vi "tipshaping.action.vi"(8 "Error in (no error)":errorcluster, 10 "Application reference":refnum<vi>, 11 "TipShapingParam":T1={"TipLift"=-1.8e-09, "Bias Settling Time"=0.2, "Lift Height"=-3.6e-09, "Lift Time 2"=0.2, "Lifting Bias"=0.02, "Lift Time 1"=0.2} {"Lift Time 1" min=0.02 max=600.0 format="%.2p"; "Lifting Bias" format="%.3p"; "Lift Time 2" min=0.02 max=600.0 format="%.2p"; "Lift Height" format="%.2p"; "Bias Settling Time" format="%.2p"; "TipLift" format="%.2p"}) -> (0 "error out":errorcluster, 2 "Application ref out":refnum<vi>, 3 "dz":sgl=-5.693078e-09)   [LabVIEW 2014]
uses:
  <userlib>/Nanonis Prog Interface V5/Nanonis Prog Interface.lvlib
panel:
  out "z channel":i32=30
  out "initialz":sgl=-5.016415e-08 format="%#_6p"
  in  "Feedback":bool=TRUE
  in  "Switch Gain":bool
  in  "Current Gain":u16(ring) items=["HS 10^5", "HS 10^6", "HS 10^7", "HS 10^8", "HS 10^9", "HS 10^10", "HS 10^11", "LN 10^3", "LN 10^4", "LN 10^5", "LN 10^6", "LN 10^7", "LN 10^8", "LN 10^9"]
  in  "Bias value":dbl=1.0 format="%.3p"
  in  "Change Bias":bool
  out "Lift Time 1":dbl=0.2 min=0.02 max=600.0 format="%.2p"
  in  "End Wait Time":dbl=0.1 format="%.2p"
  out "Lifting Bias":dbl=-8.0 format="%.3p"
  out "Lift Time 2":dbl=0.2 min=0.02 max=600.0 format="%.2p"
  out "Lift Height":dbl format="%.2p"
  out "Bias Settling Time":dbl=0.2 format="%.2p"
  out "TipLift":dbl format="%.2p"
  in  "Switch Off Delay":dbl=0.1 format="%.2p"
  out "allQuit":bool
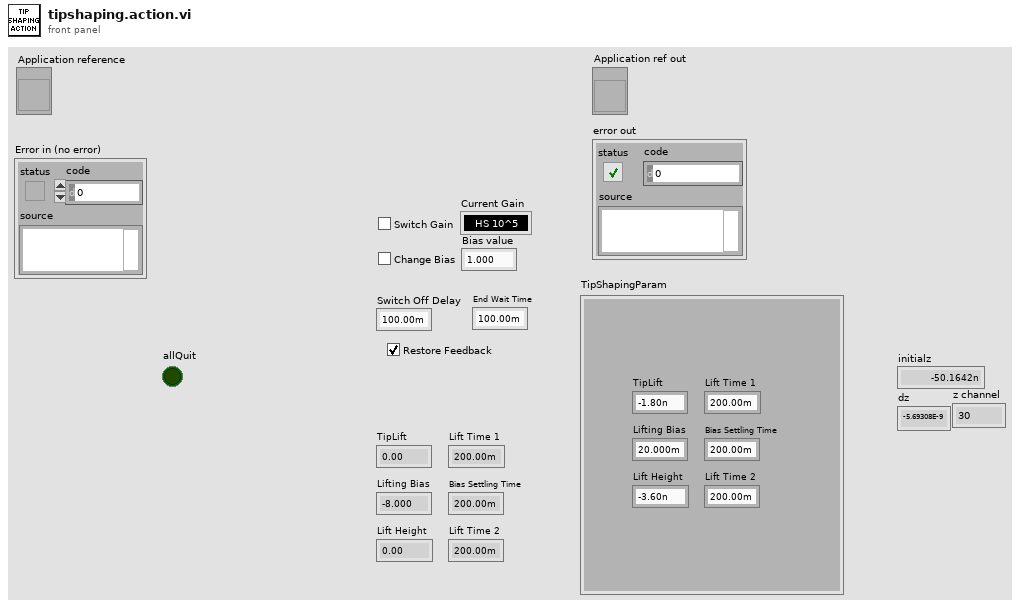
[diagram p1: front panel]
types:
  T1 = cluster{"TipLift":dbl, "Bias Settling Time":dbl, "Lift Height":dbl, "Lift Time 2":dbl, "Lifting Bias":dbl, "Lift Time 1":dbl}
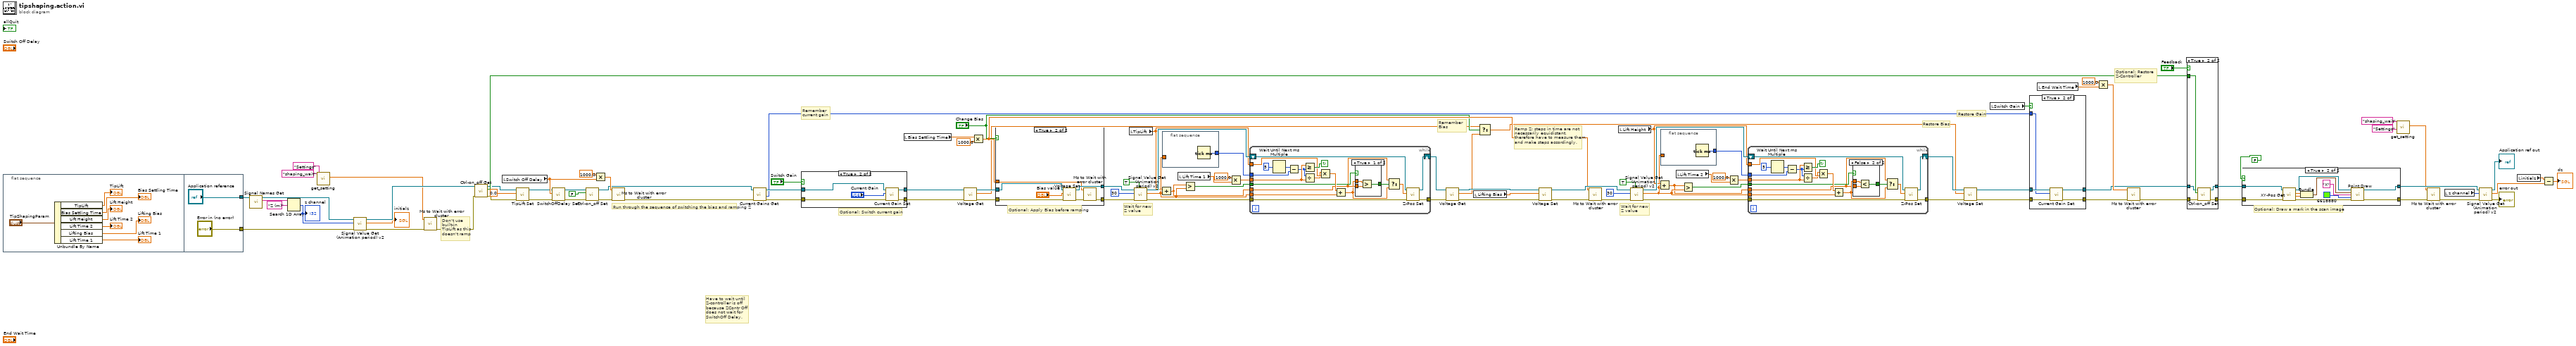
[diagram p0: block diagram]
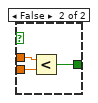
[diagram p6: hidden frame]
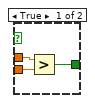
[diagram p8: hidden frame]
diagram:
  # "Ramp Z: steps in time are not necessarily equidistant, therefore have to measure them and make steps accordingly."
  # "Optional: Draw a mark in the scan image"
  # "Optional: Apply Bias before ramping"
  # "Remember Bias"
  # "Optional: Switch current gain"
  # "Remember current gain"
  # "Restore Bias"
  # "Optional: Restore Z-Controller"
  # "Restore Gain"
  # "Don't use built-in TipLift as this doesn't ramp"
  # "Wait for new Z value"
  # "Have to wait until Z-controller is off because ZContr Off does not wait for SwitchOff Delay."
  # "Wait for new Z value"
  # "Run through the sequence of switching the bias and ramping Z"
  n1 = flat-sequence {
    tunnel: ["Application reference"] -> w15
    tunnel: ["Error in (no error)"] -> w14
    frame #0 {
      n2 = Unbundle By Name("TipShapingParam") -> ("TipLift"=→"TipLift":dbl, "Bias Settling Time"=→"Bias Settling Time":dbl, "Lift Height"=→"Lift Height":dbl, "Lift Time 2"=→"Lift Time 2":dbl, "Lifting Bias"=→"Lifting Bias":dbl, "Lift Time 1"=→"Lift Time 1":dbl)
    }
    frame #1 {
    }
  }
  n3 = call <userlib>:"Signal Names Get.vi"("Application ref in"=w15) -> ("Signals Names"=w20:string[], "Application ref out"=w17:refnum<vi>)  [unwired: 6 in, 1 out]
  n4 = Search 1D Array(1D array=w20, element="Z (m)") -> (index of element=w18:i32)  [unwired: 1 in]
  "z channel" <- w18
  n5 = call "get_setting.vi"("section"="Settings", "key"="shaping_wait") -> ("output 1"=w2:dbl)  [unwired: 5 in, 4 out]
  n6 = call <userlib>:"Signal Value Get (Animation period) v2.vi"("error in (no error)"=w14, "Signal index (0-79)"=w18, "Application ref in"=w17) -> ("error out"=w9:errorcluster, "Signal value"=→"initialz":sgl, "Application ref out"=w26:refnum<vi>)  [unwired: 5 in]
  n7 = call <userlib>:"Ms to Wait with error cluster.vi"("error in (no error)"=w9, "milliseconds to wait"=w2) -> ("error out"=w8:errorcluster)  [unwired: 4 in, 1 out]
  n8 = call <userlib>:"Ctrl-on_off Get.vi"("error in (no error)"=w8, "Application ref in"=w26) -> ("error out"=w85:errorcluster, "Z-Controller on/off status"=w84:bool, "Application ref out"=w69:refnum<vi>)  [unwired: 7 in]
  n9 = local read "Switch Off Delay"() -> (w93:dbl)
  n10 = call <userlib>:"TipLift Set.vi"("error in (no error)"=w85, "TipLift (m)"=sgl 0.0, "Application ref in"=w69) -> ("error out"=w104:errorcluster, "Application ref out"=w68:refnum<vi>)  [unwired: 7 in]
  n11 = call <userlib>:"SwitchOffDelay Set.vi"("error in (no error)"=w104, "Switch off Delay (s)"=w93, "Application ref in"=w68) -> ("error out"=w75:errorcluster, "Application ref out"=w67:refnum<vi>)  [unwired: 7 in]
  n12 = call <userlib>:"Ctrl-on_off Set.vi"("error in (no error)"=w75, "Z Controller ON/OFF"=FALSE, "Application ref in"=w67) -> ("error out"=w89:errorcluster, "Application ref out"=w44:refnum<vi>)  [unwired: 7 in]
  n13 = Multiply(x=1000.0, y=w93) -> (x*y=w83:dbl)
  n14 = call <userlib>:"Ms to Wait with error cluster.vi"("error in (no error)"=w89, "milliseconds to wait"=w83) -> ("error out"=w42:errorcluster)  [unwired: 4 in, 1 out]
  n15 = call <userlib>:"Current Gains Get.vi"("Error in (no error)"=w42, "Application ref in"=w44) -> ("Error out"=w41:errorcluster, "Selected Gain"=w35:u16, "Application ref out"=w43:refnum<vi>)  [unwired: 6 in, 1 out]
  n16 = case shown="True" "Switch Gain" {
    tunnel: w43 -> [w115 w120]
    tunnel: w41 -> [w114 w119]
    tunnel: [w115 w117] -> w49
    tunnel: [w114 w118] -> w47
    frame False {
    }
    frame True {
      n17 = call <userlib>:"Current Gain Set.vi"("Error in (no error)"=w119, "Gain index"="Current Gain", "Application ref in"=w120) -> ("Error out"=w118:errorcluster, "Application ref out"=w117:refnum<vi>)  [unwired: 7 in]
    }
  }
  n18 = local read "Bias Settling Time"() -> (w91:dbl)
  n19 = call <userlib>:"Voltage Get.vi"("error in (no error)"=w47, "Application ref in"=w49) -> ("error out"=w46:errorcluster, "Bias (V)"=w45:sgl, "Application ref out"=w48:refnum<vi>)  [unwired: 7 in]
  n20 = Multiply(x=w91, y=1000.0) -> (x*y=w53:dbl)
  n21 = case shown="True" "Change Bias" {
    tunnel: w48 -> [w122 w124]
    tunnel: [w122 w128] -> w55
    tunnel: w46 -> [w121 w123]
    tunnel: [w121 w127] -> w54
    tunnel: w53 -> [_ w126]
    frame False {
    }
    frame True {
      n22 = call <userlib>:"Voltage Set.vi"("Error in (no error)"=w123, "Bias (V)"="Bias value", "Application ref in"=w124) -> ("Error out"=w129:errorcluster, "Application ref out"=w128:refnum<vi>)  [unwired: 7 in]
      n23 = call <userlib>:"Ms to Wait with error cluster.vi"("error in (no error)"=w129, "milliseconds to wait"=w126) -> ("error out"=w127:errorcluster)  [unwired: 4 in, 1 out]
    }
  }
  n24 = local read "TipLift"() -> (w34:dbl)
  n25 = call <userlib>:"Signal Value Get (Animation period) v2.vi"("Wait for newest data (F=False)"=TRUE ("Wait for newest data (F)"), "error in (no error)"=w54, "Signal index (0-79)"=i8 30 ("Signal index (0-23)"), "Application ref in"=w55) -> ("error out"=w78:errorcluster, "Signal value"=w32:sgl, "Application ref out"=w65:refnum<vi>)  [unwired: 4 in]
  n26 = Add(x=w34, y=w32) -> (x+y=w33:dbl)
  n27 = flat-sequence {
    tunnel: [w130] -> w77
    tunnel: w32 -> [_]
    frame #0 {
      n28 = Tick Count (ms)() -> (millisecond timer value=w130:u32)
    }
  }
  n29 = local read "Lift Time 1"() -> (w73:dbl)
  n30 = Greater?(x=w33, y=w32) -> (0:w31:bool)
  n31 = Multiply(x=1000.0, y=w73) -> (x*y=w72:dbl)
  n32 = while {
    tunnel: w77 -> [w149]
    tunnel: w34 -> [w147]
    tunnel: [w146] -> w71
    tunnel: w32 -> [w142]
    tunnel: w78 -> [w143]
    tunnel: w72 -> [w140]
    shift-right: [w136] -> w64
    shift-left: w65 -> [w137]
    tunnel: w33 -> [w133]
    tunnel: w31 -> [w135]
    stop <- w148 continue-if-true
    n33 = Wait Until Next ms Multiple(millisecond multiple=u32 5) -> (millisecond timer value=w139:u32)
    n34 = Subtract(x=w139, y=w149) -> (x-y=w138:u32)
    n35 = Greater Or Equal?(x=w140, y=w138) -> (x >= y?=w148:bool)
    n36 = Divide(x=w138, y=w140) -> (x/y=w144:dbl)
    n37 = Multiply(x=w144, y=w147) -> (x*y=w141:dbl)
    n38 = Add(x=w141, y=w142) -> (x+y=w132:dbl)
    n39 = case shown="True" w135 {
      tunnel: w132 -> [w152 w155]
      tunnel: w133 -> [w151 w154]
      tunnel: [w150 w153] -> w134
      frame True {
        n40 = Greater?(x=w152, y=w151) -> (0:w150:bool)
      }
      frame False {
        n41 = Less?(x=w155, y=w154) -> (x < y?=w153:bool)
      }
    }
    n42 = Select(t=w133, s=w134, f=w132) -> (s? t:f=w131:dbl)
    n43 = call <userlib>:"Z-Pos Set.vi"("error in (no error)"=w143, "Z position (m)"=w131, "Application ref in"=w137) -> ("error out"=w146:errorcluster, "Application ref out"=w136:refnum<vi>)  [unwired: 7 in]
  }
  n44 = call <userlib>:"Voltage Get.vi"("error in (no error)"=w71, "Application ref in"=w64) -> ("error out"=w70:errorcluster, "Bias (V)"=w51:sgl, "Application ref out"=w63:refnum<vi>)  [unwired: 7 in]
  n45 = local read "Lifting Bias"() -> (w103:dbl)
  n46 = Select(t=w45, s="Change Bias", f=w51) -> (s? t:f=w50:sgl)
  n47 = call <userlib>:"Voltage Set.vi"("Error in (no error)"=w70, "Bias (V)"=w103, "Application ref in"=w63) -> ("Error out"=w88:errorcluster, "Application ref out"=w59:refnum<vi>)  [unwired: 7 in]
  n48 = call <userlib>:"Ms to Wait with error cluster.vi"("error in (no error)"=w88, "milliseconds to wait"=w53) -> ("error out"=w82:errorcluster)  [unwired: 4 in, 1 out]
  n49 = local read "Lift Height"() -> (w30:dbl)
  n50 = call <userlib>:"Signal Value Get (Animation period) v2.vi"("Wait for newest data (F=False)"=TRUE ("Wait for newest data (F)"), "error in (no error)"=w82, "Signal index (0-79)"=i8 30 ("Signal index (0-23)"), "Application ref in"=w59) -> ("error out"=w81:errorcluster, "Signal value"=w29:sgl, "Application ref out"=w61:refnum<vi>)  [unwired: 4 in]
  n51 = Add(x=w30, y=w29) -> (x+y=w27:dbl)
  n52 = flat-sequence {
    tunnel: [w156] -> w97
    tunnel: w29 -> [_]
    frame #0 {
      n53 = Tick Count (ms)() -> (millisecond timer value=w156:u32)
    }
  }
  n54 = local read "Lift Time 2"() -> (w101:dbl)
  n55 = Greater?(x=w27, y=w29) -> (0:w28:bool)
  n56 = Multiply(x=1000.0, y=w101) -> (x*y=w90:dbl)
  n57 = while {
    tunnel: w97 -> [w175]
    tunnel: w30 -> [w173]
    tunnel: [w172] -> w99
    tunnel: w29 -> [w168]
    tunnel: w81 -> [w169]
    tunnel: w90 -> [w166]
    shift-right: [w162] -> w60
    shift-left: w61 -> [w163]
    tunnel: w28 -> [w161]
    tunnel: w27 -> [w158]
    stop <- w174 continue-if-true
    n58 = Wait Until Next ms Multiple(millisecond multiple=u32 5) -> (millisecond timer value=w165:u32)
    n59 = Subtract(x=w165, y=w175) -> (x-y=w164:u32)
    n60 = Greater Or Equal?(x=w166, y=w164) -> (x >= y?=w174:bool)
    n61 = Divide(x=w164, y=w166) -> (x/y=w170:dbl)
    n62 = Multiply(x=w170, y=w173) -> (x*y=w167:dbl)
    n63 = Add(x=w167, y=w168) -> (x+y=w159:dbl)
    n64 = case shown="False" w161 {
      tunnel: w159 -> [w178 w181]
      tunnel: w158 -> [w177 w180]
      tunnel: [w176 w179] -> w160
      frame True {
        n65 = Greater?(x=w178, y=w177) -> (0:w176:bool)
      }
      frame False {
        n66 = Less?(x=w181, y=w180) -> (x < y?=w179:bool)
      }
    }
    n67 = Select(t=w158, s=w160, f=w159) -> (s? t:f=w157:dbl)
    n68 = call <userlib>:"Z-Pos Set.vi"("error in (no error)"=w169, "Z position (m)"=w157, "Application ref in"=w163) -> ("error out"=w172:errorcluster, "Application ref out"=w162:refnum<vi>)  [unwired: 7 in]
  }
  n69 = call <userlib>:"Voltage Set.vi"("Error in (no error)"=w99, "Bias (V)"=w50, "Application ref in"=w60) -> ("Error out"=w37:errorcluster, "Application ref out"=w39:refnum<vi>)  [unwired: 7 in]
  n70 = local read "Switch Gain"() -> (w40:bool)
  n71 = case shown="True" w40 {
    tunnel: w39 -> [w183 w188]
    tunnel: [w183 w187] -> w38
    tunnel: w37 -> [w182 w186]
    tunnel: [w182 w185] -> w36
    tunnel: w35 -> [_ w184]
    frame False {
    }
    frame True {
      n72 = call <userlib>:"Current Gain Set.vi"("Error in (no error)"=w186, "Gain index"=w184, "Application ref in"=w188) -> ("Error out"=w185:errorcluster, "Application ref out"=w187:refnum<vi>)  [unwired: 7 in]
    }
  }
  n73 = local read "End Wait Time"() -> (w95:dbl)
  n74 = Multiply(x=1000.0, y=w95) -> (x*y=w86:dbl)
  n75 = call <userlib>:"Ms to Wait with error cluster.vi"("error in (no error)"=w36, "milliseconds to wait"=w86) -> ("error out"=w87:errorcluster)  [unwired: 4 in, 1 out]
  n76 = case shown="True" "Feedback" {
    tunnel: w87 -> [w189 w195]
    tunnel: w84 -> [_ w194]
    tunnel: w38 -> [w190 w193]
    tunnel: [w190 w192] -> w58
    tunnel: [w189 w191] -> w57
    frame False {
    }
    frame True {
      n77 = call <userlib>:"Ctrl-on_off Set.vi"("error in (no error)"=w195, "Z Controller ON/OFF"=w194, "Application ref in"=w193) -> ("error out"=w191:errorcluster, "Application ref out"=w192:refnum<vi>)  [unwired: 7 in]
    }
  }
  n78 = case shown="True" FALSE {
    tunnel: w58 -> [w196 w207]
    tunnel: w57 -> [_ w205]
    tunnel: [w196 w203] -> w25
    tunnel: [_ w197] -> w11
    frame False {
    }
    frame True {
      n79 = call <userlib>:"XY-Pos Get.vi"("error in (no error)"=w205, "Application ref in"=w207) -> ("error out"=w204:errorcluster, "Y (m)"=w201:sgl, "X (m)"=w202:sgl, "Application ref out"=w206:refnum<vi>)  [unwired: 5 in]
      n80 = Bundle("X (m)"=w202, "Y (m)"=w201) -> (w200:cluster{"X (m)":sgl, "Y (m)":sgl})  [unwired: 1 in]
      n81 = call <userlib>:"Point Draw.vi"("Application ref in"=w206, "Point Coordinates"=w200, "Text"="X", "Color"=u32 6618880, "error in (no error)"=w204) -> ("Application ref out"=w203:refnum<vi>, "error out"=w197:errorcluster)  [unwired: 9 in]
    }
  }
  n82 = call "get_setting.vi"("section"="Settings", "key"="shaping_wait") -> ("output 1"=w5:dbl)  [unwired: 5 in, 4 out]
  n83 = call <userlib>:"Ms to Wait with error cluster.vi"("error in (no error)"=w11, "milliseconds to wait"=w5) -> ("error out"=w10:errorcluster)  [unwired: 4 in, 1 out]
  n84 = local read "z channel"() -> (w16:i32)
  n85 = call <userlib>:"Signal Value Get (Animation period) v2.vi"("error in (no error)"=w10, "Signal index (0-79)"=w16, "Application ref in"=w25) -> ("error out"=→"error out":errorcluster, "Signal value"=w22:sgl, "Application ref out"=→"Application ref out":refnum<vi>)  [unwired: 5 in]
  n86 = local read "initialz"() -> (w23:sgl)
  n87 = Subtract(x=w23, y=w22) -> (x-y=→"dz":sgl)
